vi "UDPSender.vi"(9 "Action":enum16{"Send", "Initialize", "Close"}(ring), 11 "Pod Monitoring Telemetry":string) -> (0 "error out":errorcluster)   [LabVIEW 2017]
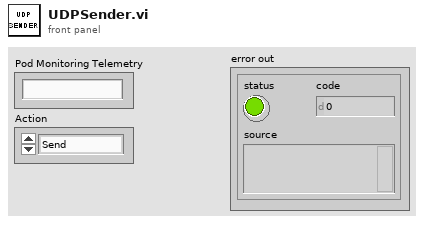
[diagram p1: front panel]
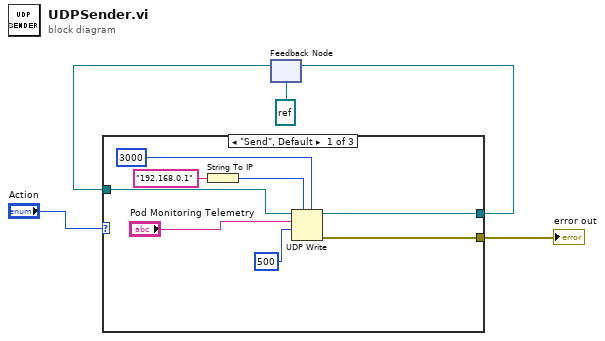
[diagram p0: block diagram]
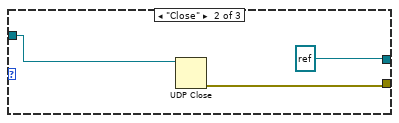
[diagram p2: hidden frame]
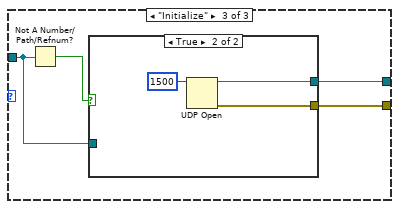
[diagram p3: hidden frame]
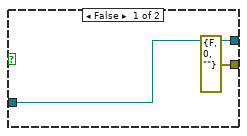
[diagram p4: hidden frame]
diagram:
  n1 = feedback #1(refnum<k16> refnum ("port")) -> (w2:refnum<k16>)
  n2 = case shown="\"Send\", Default" "Action" {
    tunnel: [w8 refnum<k16> refnum ("port") w20] -> w4
    tunnel: w2 -> [w13 w16 w18]
    tunnel: [w7 w15 w17] -> w1
    frame "Send", Default {
      n3 = String To IP(1:"192.168.0.1" ("name")) -> (0:w11:u32)
      n4 = UDP Write(address=w11, port or service name=u16 3000, connection ID=w13, data in="Pod Monitoring Telemetry", 9:500 ("timeout ms (25000)")) -> (error out=w7:errorcluster, 3:w8:refnum<k16>)  [unwired: 1 in]
    }
    frame "Close" {
      n5 = UDP Close(connection ID=w16) -> (error out=w15:errorcluster)  [unwired: 1 in, 1 out]
    }
    frame "Initialize" {
      n6 = Not A Number/Path/Refnum?(number/path/refnum=w18) -> (NaN/Path/Refnum?=w19:bool)
      n7 = case shown="True" w19 {
        tunnel: [w22 w25] -> w20
        tunnel: w18 -> [w22 _]
        tunnel: [errorcluster {"status"=FALSE, "code"=0, "source"=""} ("error out") w23] -> w17
        frame False {
        }
        frame True {
          n8 = UDP Open(11:u16 1500 ("port")) -> (port=w25:refnum<k16>, 0:w23:errorcluster)  [unwired: 4 in, 1 out]
        }
      }
    }
  }
  "error out" <- w1
  n9 = feedback-in #1(w4) -> ()
